vi "Initialize.vi"(5 "Dictionary File Path":path, 11 "error in":errorcluster) -> (2 "CSV String":string, 4 "Dictionary":T1, 6 "Dictionary File Path out":path, 8 "Languages":string[](array[string]), 10 "Current Language":string, 15 "error out":errorcluster)   [LabVIEW 2020]
doc: "Loads the language dictionary from file.\n\nReturns the current language (defined by the OS), and available languages in the dictionary."
uses:
  SubVIs/Dictionary--Cluster.ctl
  SubVIs/Font -- Cluster.ctl
  SubVIs/Phrase Dictionary Entry -- Cluster.ctl
  SubVIs/Localization FGV Action -- Enum.ctl
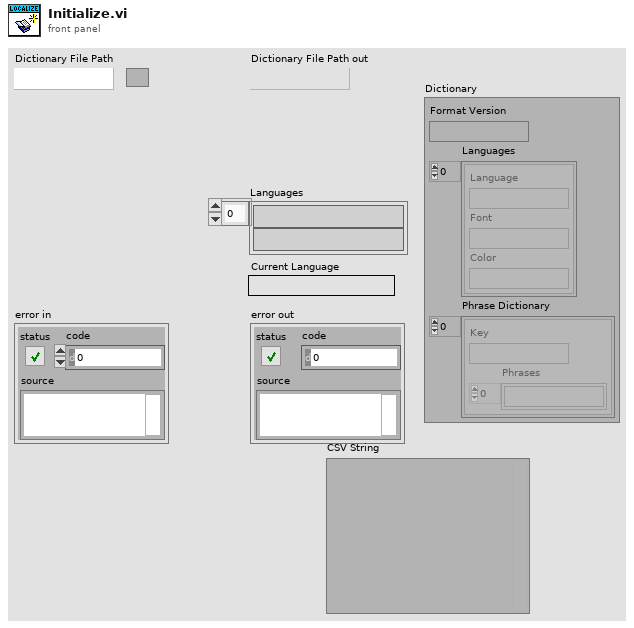
[diagram p1: front panel]
types:
  T1 = typedef "Dictionary--Cluster.ctl" = cluster{"Format Version":string, "Languages":T2[], "Phrase Dictionary":T3[]}
  T2 = typedef "Font -- Cluster.ctl" = cluster{"Language":string, "Font":string, "Color":string}
  T3 = typedef "Phrase Dictionary Entry -- Cluster.ctl" = cluster{"Key":string, "Phrases":string[]}
  T4 = typedef "Localization FGV Action -- Enum.ctl" = enum16{"Read Dictionary", "Translate VIs", "Register VI", "Get Languages", "Translate Phrase", "Get Key For Phrase", "Get Phrase For Phrase", "Translate VI", "Unregister"}
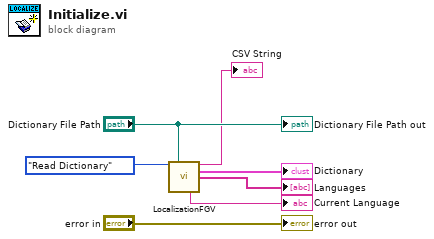
[diagram p0: block diagram]
diagram:
  n1 = call "LocalizationFGV.vi"("Action"=Localization_FGV_Action_--_Enum."Read Dictionary", "Dictionary File Path"="Dictionary File Path") -> ("CSV String"=→"CSV String":string, "Dictionary"=→"Dictionary":T1, "Languages"=→"Languages":string[], "Current Language"=→"Current Language":string)  [unwired: 8 in, 2 out]
  "Dictionary File Path out" <- "Dictionary File Path"
  "error out" <- "error in"
